vi "Read_Image.vi"(6 "PreProcessing_Options":T2={"Image Type"=4, "Normalization Type"=enum."Standardize(DS_Stats)", "Interpolation Type"=1} {"Interpolation Type" items=["Zero Order", "Bi-Linear", "Quadratic", "Cubic Spline"]; "Image Type" items=["Grayscale (U8)", "Grayscale (I16)", "Grayscale (SGL)", "Complex (CSG)", "RGB (U32)", "HSL (U32)", "RGB (U64)", "Grayscale (U16)"]}, 7 "Dataset_Stats":T5={"means"={"R"=0.5385, "G"=0.5348, "B"=0.551}, "vars"={"R"=0.3673, "G"=0.3673, "B"=0.3505}, "DS_Size"=0} {"vars"."R" format="%#_3g"; "vars"."G" format="%#_3g"; "vars"."B" format="%#_3g"; "means"."R" format="%#_3g"; "means"."G" format="%#_3g"; "means"."B" format="%#_3g"}, 8 "error in":errorcluster, 10 "Target_Dims":T1={"C"=3, "H"=224, "W"=224}, 11 "Img Path":path=path "D:/DNN/MVTec/bottle/test/good/019.png") -> (0 "error out":errorcluster, 3 "Image Out":sgl[][][](array[numeric]), 5 "dT_Img_Read":dbl=0.026547699992079288 format="%#_6p")   [LabVIEW 2020]
uses:
  PatchCore_AddOn/API/Controls/NNPC_DS_Stats.ctl
  PatchCore_AddOn/API/Controls/Image_Stats_RGB.ctl
  Controls/ImRead_PreProcessing_Options.ctl
  PatchCore_AddOn/Low_Level/Controls/Normalization_Type.ctl
  <vilib>/Ngene/Deep Learning Toolkit/Toolkit/NN_Data/API/NN_Dims(C,H,W).ctl
  63923816-9007-4586-bbbc-381e18ed1900.vi
  9c50cdeb-22e2-48bb-a9e5-933b6d93635b.vi
  <vilib>/vision/NI_Vision_Development_Module.lvlib
  PatchCore_AddOn/PatchCore_AddOn.lvlib
  <vilib>/Ngene/Deep Learning Toolkit/Toolkit/Deep_Learning_Toolkit_by_Ngene.lvlib
panel:
  out "dT_Image_Read(IMAQ)":dbl=0.0232819999800995 format="%#_6p"
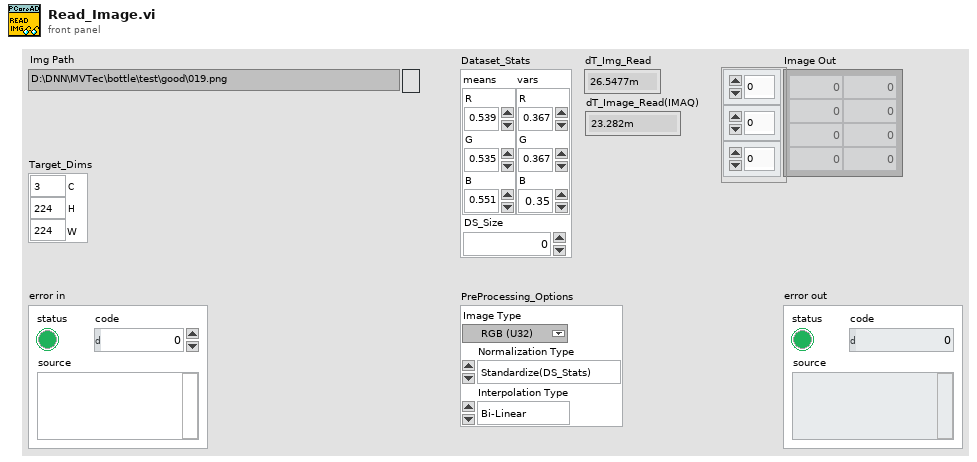
[diagram p1: front panel]
types:
  T1 = typedef "Deep_Learning_Toolkit_by_Ngene.lvlib/NN_Dims(C,H,W).ctl" = cluster{"C":i32, "H":i32, "W":i32}
  T2 = typedef "ImRead_PreProcessing_Options.ctl" = cluster{"Image Type":T3, "Normalization Type":T4, "Interpolation Type":u32}
  T3 = typedef "Image Type" = u32
  T4 = typedef "PatchCore_AddOn.lvlib/Normalization_Type.ctl" = enum16{"Standardize(DS_Stats)", "Standardize(Image_Stats)"}
  T5 = typedef "PatchCore_AddOn.lvlib/NNPC_DS_Stats.ctl" = cluster{"means":T6, "vars":T6, "DS_Size":i32}
  T6 = typedef "PatchCore_AddOn.lvlib/Image_Stats_RGB.ctl" = cluster{"R":sgl, "G":sgl, "B":sgl}
  T7 = typedef "IMAQ Image.ctl" = refnum<image>
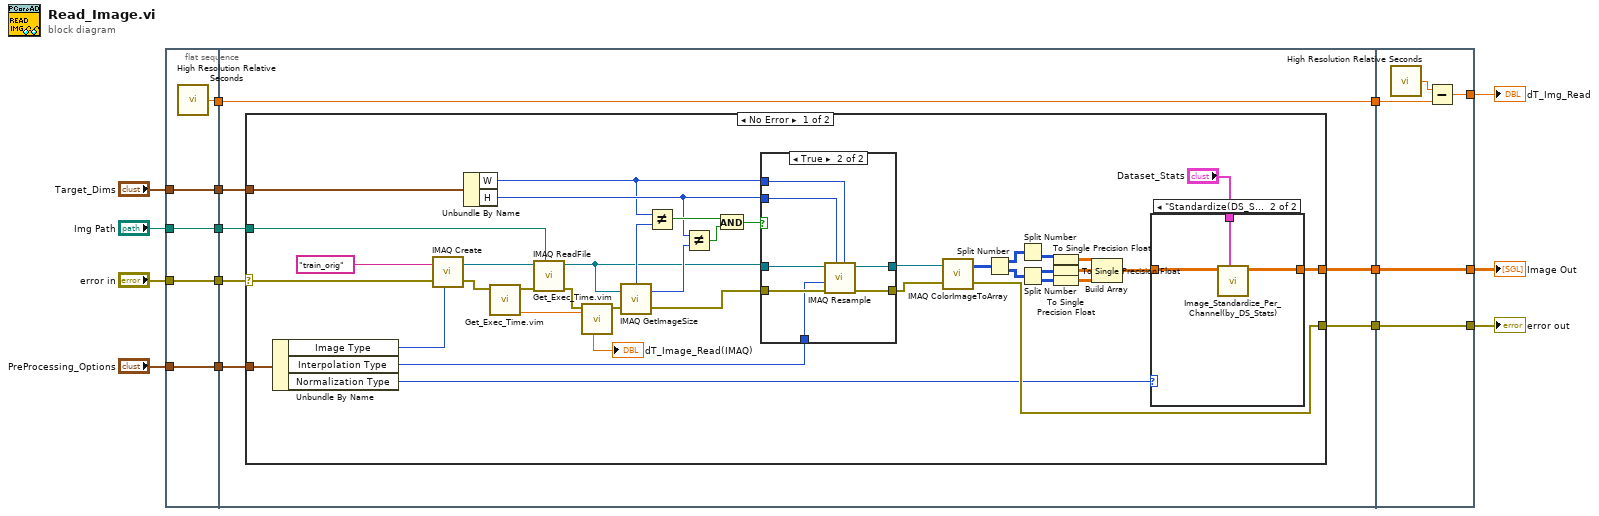
[diagram p0: block diagram]
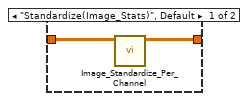
[diagram p2: hidden frame]
diagram:
  n1 = flat-sequence {
    tunnel: [w20] -> w15
    tunnel: "Img Path" -> [w19]
    tunnel: [w19] -> w12
    tunnel: [w18] -> w10
    tunnel: "error in" -> [w18]
    tunnel: [w17] -> w5
    tunnel: "PreProcessing_Options" -> [w17]
    tunnel: [w16] -> w3
    tunnel: "Target_Dims" -> [w16]
    tunnel: [w27] -> w14
    tunnel: w15 -> [w27]
    tunnel: w12 -> [w26]
    tunnel: w10 -> [w23]
    tunnel: [w25] -> w8
    tunnel: [w24] -> w7
    tunnel: w5 -> [w22]
    tunnel: w3 -> [w21]
    tunnel: w14 -> [w85]
    tunnel: [w84] -> w13
    tunnel: [w83] -> w1
    tunnel: w8 -> [w83]
    tunnel: [w82] -> w6
    tunnel: w7 -> [w82]
    frame #0 {
      n2 = call <vilib>:"High Resolution Relative Seconds.vi"() -> ("relative seconds"=w20:dbl)
    }
    frame #1 {
      n3 = case shown="No Error" w23 {
        selector: w23 -> [w54 w81]
        tunnel: w26 -> [w64 _]
        tunnel: [w56 _] -> w25
        tunnel: [w55 w81] -> w24
        tunnel: w22 -> [w34 _]
        tunnel: w21 -> [w30 _]
        frame No Error {
          n4 = Unbundle By Name(w34) -> ("Image Type"=w33:T3, "Interpolation Type"=w31:u32, "Normalization Type"=w32:T4)
          n5 = call "IMAQ Create"("Image Name"="train_orig", "Image Type"=w33, "error in (no error)"=w54) -> ("New Image"=w66:T7, "error out"=w49:errorcluster)  [unwired: 2 in]
          n6 = Unbundle By Name(w30) -> ("W"=w51:i32, "H"=w52:i32)
          n7 = call "Get_Exec_Time.vim"("error in (no error)"=w49) -> ("T(n)"=w45:dbl, "error out"=w47:errorcluster)  [unwired: 6 in, 1 out]
          n8 = call "IMAQ ReadFile"("File Path"=w64, "error in (no error)"=w47, "Image"=w66) -> ("error out"=w50:errorcluster, "Image Out"=w28:T7)  [unwired: 4 in, 3 out]
          n9 = call "Get_Exec_Time.vim"("T(n-1)"=w45, "error in (no error)"=w50) -> ("error out"=w46:errorcluster, "dT"=→"dT_Image_Read(IMAQ)":dbl)  [unwired: 5 in, 1 out]
          n10 = call "IMAQ GetImageSize"("Image"=w28, "error in (no error)"=w46) -> ("Y Resolution"=w62:i32, "X Resolution"=w63:i32, "error out"=w58:errorcluster)  [unwired: 2 in]
          n11 = Not Equal?(x=w51, y=w63) -> (x != y?=w60:bool)
          n12 = Not Equal?(x=w52, y=w62) -> (x != y?=w61:bool)
          n13 = And(x=w60, y=w61) -> (x .and. y?=w59:bool)
          n14 = case shown="True" w59 {
            tunnel: w51 -> [_ w80]
            tunnel: w52 -> [_ w79]
            tunnel: [w72 w77] -> w53
            tunnel: [w73 w78] -> w48
            tunnel: w58 -> [w73 w76]
            tunnel: w28 -> [w72 w75]
            tunnel: w31 -> [_ w74]
            frame False {
            }
            frame True {
              n15 = call "IMAQ Resample"("X Resolution"=w80, "Y Resolution"=w79, "error in (no error)"=w76, "Interpolation Type"=w74, "Image Src"=w75) -> ("error out"=w78:errorcluster, "Image Dst Out"=w77:T7)  [unwired: 5 in]
            }
          }
          n16 = call "IMAQ ColorImageToArray"("Image"=w53, "error in (no error)"=w48) -> ("Image Pixels (U32)"=w57:u32[][], "error out"=w55:errorcluster)  [unwired: 2 in, 1 out]
          n17 = Split Number(x=w57) -> (hi(x)=w42:u16[][], lo(x)=w43:u16[][])
          n18 = Split Number(x=w42) -> (lo(x)=w41:u8[][])  [unwired: 1 out]
          n19 = Split Number(x=w43) -> (hi(x)=w40:u8[][], lo(x)=w39:u8[][])
          n20 = To Single Precision Float(number=w41) -> (single precision float=w38:sgl[][])
          n21 = To Single Precision Float(number=w40) -> (single precision float=w37:sgl[][])
          n22 = To Single Precision Float(number=w39) -> (single precision float=w36:sgl[][])
          n23 = Build Array(w38, w37, w36) -> (w29:sgl[][][])
          n24 = case shown="\"Standardize(DS_Stats)\"" w32 {
            tunnel: w29 -> [w68 w71]
            tunnel: [w67 w70] -> w56
            tunnel: "Dataset_Stats" -> [_ w69]
            frame "Standardize(Image_Stats)", Default {
              n25 = call "Image_Standardize_Per_Channel.vi"("Input 3D"=w68) -> ("Normalized"=w67:sgl[][][])  [unwired: 10 in]
            }
            frame "Standardize(DS_Stats)" {
              n26 = call "Image_Standardize_Per_Channel(by_DS_Stats).vi"("Dataset_Stats"=w69, "In"=w71) -> ("Out"=w70:sgl[][][])  [unwired: 9 in]
            }
          }
        }
        frame Error {
        }
      }
    }
    frame #2 {
      n27 = call <vilib>:"High Resolution Relative Seconds.vi"() -> ("relative seconds"=w86:dbl)
      n28 = Subtract(x=w86, y=w85) -> (x-y=w84:dbl)
    }
  }
  "dT_Img_Read" <- w13
  "Image Out" <- w1
  "error out" <- w6
